vi "for_v0_v30.vi"() -> ()   [LabVIEW 2009]
panel:
  in  "stop":bool
  out "Picture":picture
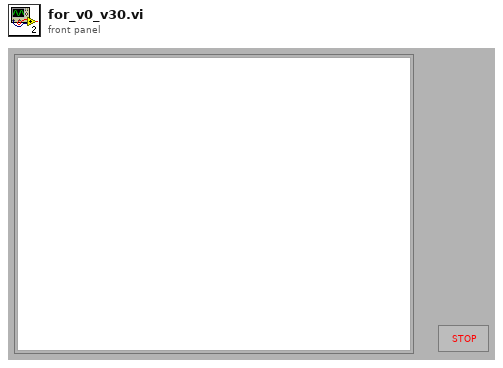
[diagram p1: front panel]
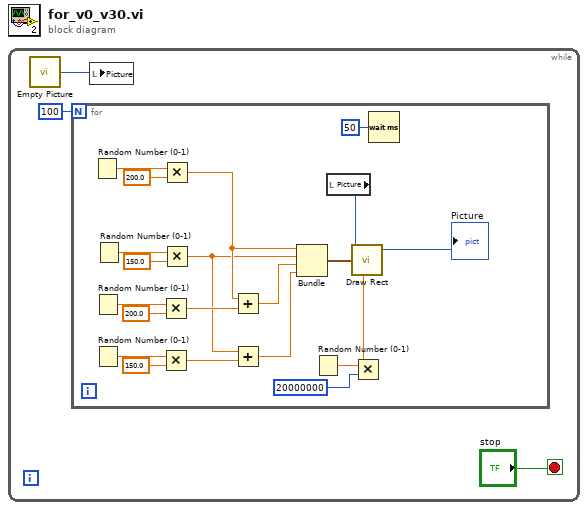
[diagram p0: block diagram]
diagram:
  n1 = while {
    stop <- "stop" stop-if-true
    n2 = call "Empty Picture"() -> ("empty picture"=w2:picture)
    n3 = for {
      N: 100 -> [_]
      n4 = Random Number (0-1)() -> (number: 0 to 1=w20:dbl)
      n5 = Random Number (0-1)() -> (number: 0 to 1=w16:dbl)
      n6 = Random Number (0-1)() -> (number: 0 to 1=w14:dbl)
      n7 = Random Number (0-1)() -> (number: 0 to 1=w19:dbl)
      n8 = Multiply(x=w16, y=200.0) -> (x*y=w11:dbl)
      n9 = Multiply(x=w14, y=150.0) -> (x*y=w8:dbl)
      n10 = Multiply(x=w20, y=200.0) -> (x*y=w12:dbl)
      n11 = Multiply(x=w19, y=150.0) -> (x*y=w9:dbl)
      n12 = Add(x=w12, y=w11) -> (x+y=w10:dbl)
      n13 = Add(x=w9, y=w8) -> (x+y=w7:dbl)
      n14 = Bundle(w12, w9, w10, w7) -> (w23:cluster{dbl, dbl, dbl, dbl})  [unwired: 1 in]
      n15 = Random Number (0-1)() -> (number: 0 to 1=w6:dbl)
      n16 = local read "Picture"() -> (w24:picture)
      n17 = Multiply(x=w6, y=20000000) -> (x*y=w4:dbl)
      n18 = call <vilib>:"Draw Rect.vi"("picture"=w24, "rect"=w23, "color(black)"=w4) -> ("new picture"=→"Picture":picture)  [unwired: 6 in]
      n19 = Wait (ms)(milliseconds to wait=u32 50) -> ()  [unwired: 1 out]
    }
    n20 = local write "Picture"(w2) -> ()
  }
